vi "Lab Panel V5.0.vi"() -> ()   [LabVIEW 2013] (continued)
                      tunnel: w2173 -> [w2180 _]
                      tunnel: w2172 -> [w2179 _]
                      tunnel: w2171 -> [w2178 _]
                      frame True {
                        n1199 = stacked-sequence {
                          tunnel: w2180 -> [w2183 _]
                          tunnel: w2179 -> [_ w2188]
                          tunnel: w2178 -> [w2181 _]
                          frame #0 {
                            n1200 = Build Array("T-RISE") -> (w2185:string[])
                            n1201 = Build Array(w2183) -> (w2184:dbl[])
                            n1202 = TDMS Write(0:w2181, 5:"TEST PASS", 7:w2185, 9:w2184) -> (15:w2187:errorcluster)  [unwired: 2 in, 3 out]
                            n1203 = local write "data file error"(w2187) -> ()
                          }
                          frame #1 {
                            n1204 = Bundle(cluster=w2188, "STATUS"="T-RISE PASS") -> (w2190:T4)  [unwired: 2 in]
                            n1205 = local write "RESULT LAB01-1"(TRUE) -> ()
                            n1206 = local write "DISP LAB01-1"(w2190) -> ()
                          }
                        }
                      }
                      frame False {
                      }
                    }
                  }
                }
              }
              frame #1 {
                # "LAB01-2"
                n1207 = Equal?(x=w2193, y=2) -> (x = y?=w2196:bool)
                n1208 = local read "DISP LAB01-2"() -> (w2198:T4)
                n1209 = Unbundle(w2198) -> ("STATUS"=w2199:string)  [unwired: 2 out]
                n1210 = Equal?(x=w2199, y="RUN") -> (x = y?=w2195:bool)
                n1211 = And(x=w2195, y=w2196) -> (x .and. y?=w2194:bool)
                n1212 = case shown="True" w2194 {
                  tunnel: w2198 -> [_ w2202]
                  tunnel: w2192 -> [_ w2205]
                  frame False {
                  }
                  frame True {
                    n1213 = local read "SET LAB01-2"() -> (w2204:T5)
                    n1214 = local read "TDMS LAB01-2"() -> (w2201:refnum<k34>)
                    n1215 = Unbundle(w2202) -> ("CYCLE"=w2206:dbl)  [unwired: 2 out]
                    n1216 = Unbundle(w2204) -> ("T-RISE mins"=w2203:dbl)  [unwired: 4 out]
                    n1217 = Greater Or Equal?(x=w2206, y=w2205) -> (x >= y?=w2207:bool)
                    n1218 = case shown="True" w2207 {
                      tunnel: w2203 -> [w2210 _]
                      tunnel: w2202 -> [w2209 _]
                      tunnel: w2201 -> [w2208 _]
                      frame True {
                        n1219 = stacked-sequence {
                          tunnel: w2210 -> [w2213 _]
                          tunnel: w2209 -> [_ w2218]
                          tunnel: w2208 -> [w2211 _]
                          frame #0 {
                            n1220 = Build Array("T-RISE") -> (w2215:string[])
                            n1221 = Build Array(w2213) -> (w2214:dbl[])
                            n1222 = TDMS Write(0:w2211, 5:"TEST PASS", 7:w2215, 9:w2214) -> (15:w2217:errorcluster)  [unwired: 2 in, 3 out]
                            n1223 = local write "data file error"(w2217) -> ()
                          }
                          frame #1 {
                            n1224 = Bundle(cluster=w2218, "STATUS"="T-RISE PASS") -> (w2220:T4)  [unwired: 2 in]
                            n1225 = local write "RESULT LAB01-2"(TRUE) -> ()
                            n1226 = local write "DISP LAB01-2"(w2220) -> ()
                          }
                        }
                      }
                      frame False {
                      }
                    }
                  }
                }
              }
              frame #2 {
                # "LAB02-1"
                n1227 = Equal?(x=w2223, y=2) -> (x = y?=w2226:bool)
                n1228 = local read "DISP LAB02-1"() -> (w2228:T4)
                n1229 = Unbundle(w2228) -> ("STATUS"=w2229:string)  [unwired: 2 out]
                n1230 = Equal?(x=w2229, y="RUN") -> (x = y?=w2225:bool)
                n1231 = And(x=w2225, y=w2226) -> (x .and. y?=w2224:bool)
                n1232 = case shown="True" w2224 {
                  tunnel: w2228 -> [_ w2232]
                  tunnel: w2222 -> [_ w2235]
                  frame False {
                  }
                  frame True {
                    n1233 = local read "SET LAB02-1"() -> (w2234:T5)
                    n1234 = local read "TDMS LAB02-1"() -> (w2231:refnum<k34>)
                    n1235 = Unbundle(w2232) -> ("CYCLE"=w2236:dbl)  [unwired: 2 out]
                    n1236 = Unbundle(w2234) -> ("T-RISE mins"=w2233:dbl)  [unwired: 4 out]
                    n1237 = Greater Or Equal?(x=w2236, y=w2235) -> (x >= y?=w2237:bool)
                    n1238 = case shown="True" w2237 {
                      tunnel: w2233 -> [w2240 _]
                      tunnel: w2232 -> [w2239 _]
                      tunnel: w2231 -> [w2238 _]
                      frame True {
                        n1239 = stacked-sequence {
                          tunnel: w2240 -> [w2243 _]
                          tunnel: w2239 -> [_ w2248]
                          tunnel: w2238 -> [w2241 _]
                          frame #0 {
                            n1240 = Build Array("T-RISE") -> (w2245:string[])
                            n1241 = Build Array(w2243) -> (w2244:dbl[])
                            n1242 = TDMS Write(0:w2241, 5:"TEST PASS", 7:w2245, 9:w2244) -> (15:w2247:errorcluster)  [unwired: 2 in, 3 out]
                            n1243 = local write "data file error"(w2247) -> ()
                          }
                          frame #1 {
                            n1244 = Bundle(cluster=w2248, "STATUS"="T-RISE PASS") -> (w2250:T4)  [unwired: 2 in]
                            n1245 = local write "RESULT LAB02-1"(TRUE) -> ()
                            n1246 = local write "DISP LAB02-1"(w2250) -> ()
                          }
                        }
                      }
                      frame False {
                      }
                    }
                  }
                }
              }
              frame #3 {
                # "LAB02-2"
                n1247 = Equal?(x=w2253, y=2) -> (x = y?=w2256:bool)
                n1248 = local read "DISP LAB02-2"() -> (w2258:T4)
                n1249 = Unbundle(w2258) -> ("STATUS"=w2259:string)  [unwired: 2 out]
                n1250 = Equal?(x=w2259, y="RUN") -> (x = y?=w2255:bool)
                n1251 = And(x=w2255, y=w2256) -> (x .and. y?=w2254:bool)
                n1252 = case shown="True" w2254 {
                  tunnel: w2258 -> [_ w2262]
                  tunnel: w2252 -> [_ w2265]
                  frame False {
                  }
                  frame True {
                    n1253 = local read "SET LAB02-2"() -> (w2264:T5)
                    n1254 = local read "TDMS LAB02-2"() -> (w2261:refnum<k34>)
                    n1255 = Unbundle(w2262) -> ("CYCLE"=w2266:dbl)  [unwired: 2 out]
                    n1256 = Unbundle(w2264) -> ("T-RISE mins"=w2263:dbl)  [unwired: 4 out]
                    n1257 = Greater Or Equal?(x=w2266, y=w2265) -> (x >= y?=w2267:bool)
                    n1258 = case shown="True" w2267 {
                      tunnel: w2263 -> [w2270 _]
                      tunnel: w2262 -> [w2269 _]
                      tunnel: w2261 -> [w2268 _]
                      frame True {
                        n1259 = stacked-sequence {
                          tunnel: w2270 -> [w2273 _]
                          tunnel: w2269 -> [_ w2278]
                          tunnel: w2268 -> [w2271 _]
                          frame #0 {
                            n1260 = Build Array("T-RISE") -> (w2275:string[])
                            n1261 = Build Array(w2273) -> (w2274:dbl[])
                            n1262 = TDMS Write(0:w2271, 5:"TEST PASS", 7:w2275, 9:w2274) -> (15:w2277:errorcluster)  [unwired: 2 in, 3 out]
                            n1263 = local write "data file error"(w2277) -> ()
                          }
                          frame #1 {
                            n1264 = Bundle(cluster=w2278, "STATUS"="T-RISE PASS") -> (w2280:T4)  [unwired: 2 in]
                            n1265 = local write "RESULT LAB02-2"(TRUE) -> ()
                            n1266 = local write "DISP LAB02-2"(w2280) -> ()
                          }
                        }
                      }
                      frame False {
                      }
                    }
                  }
                }
              }
              frame #4 {
                # "LAB03-1"
                n1267 = Equal?(x=w2283, y=2) -> (x = y?=w2286:bool)
                n1268 = local read "DISP LAB03-1"() -> (w2288:T4)
                n1269 = Unbundle(w2288) -> ("STATUS"=w2289:string)  [unwired: 2 out]
                n1270 = Equal?(x=w2289, y="RUN") -> (x = y?=w2285:bool)
                n1271 = And(x=w2285, y=w2286) -> (x .and. y?=w2284:bool)
                n1272 = case shown="True" w2284 {
                  tunnel: w2288 -> [_ w2292]
                  tunnel: w2282 -> [_ w2295]
                  frame False {
                  }
                  frame True {
                    n1273 = local read "SET LAB03-1"() -> (w2294:T5)
                    n1274 = local read "TDMS LAB03-1"() -> (w2291:refnum<k34>)
                    n1275 = Unbundle(w2292) -> ("CYCLE"=w2296:dbl)  [unwired: 2 out]
                    n1276 = Unbundle(w2294) -> ("T-RISE mins"=w2293:dbl)  [unwired: 4 out]
                    n1277 = Greater Or Equal?(x=w2296, y=w2295) -> (x >= y?=w2297:bool)
                    n1278 = case shown="True" w2297 {
                      tunnel: w2293 -> [w2300 _]
                      tunnel: w2292 -> [w2299 _]
                      tunnel: w2291 -> [w2298 _]
                      frame True {
                        n1279 = stacked-sequence {
                          tunnel: w2300 -> [w2303 _]
                          tunnel: w2299 -> [_ w2308]
                          tunnel: w2298 -> [w2301 _]
                          frame #0 {
                            n1280 = Build Array("T-RISE") -> (w2305:string[])
                            n1281 = Build Array(w2303) -> (w2304:dbl[])
                            n1282 = TDMS Write(0:w2301, 5:"TEST PASS", 7:w2305, 9:w2304) -> (15:w2307:errorcluster)  [unwired: 2 in, 3 out]
                            n1283 = local write "data file error"(w2307) -> ()
                          }
                          frame #1 {
                            n1284 = Bundle(cluster=w2308, "STATUS"="T-RISE PASS") -> (w2310:T4)  [unwired: 2 in]
                            n1285 = local write "RESULT LAB03-1"(TRUE) -> ()
                            n1286 = local write "DISP LAB03-1"(w2310) -> ()
                          }
                        }
                      }
                      frame False {
                      }
                    }
                  }
                }
              }
              frame #5 {
                # "LAB03-2"
                n1287 = Equal?(x=w2313, y=2) -> (x = y?=w2316:bool)
                n1288 = local read "DISP LAB03-2"() -> (w2318:T4)
                n1289 = Unbundle(w2318) -> ("STATUS"=w2319:string)  [unwired: 2 out]
                n1290 = Equal?(x=w2319, y="RUN") -> (x = y?=w2315:bool)
                n1291 = And(x=w2315, y=w2316) -> (x .and. y?=w2314:bool)
                n1292 = case shown="True" w2314 {
                  tunnel: w2318 -> [_ w2322]
                  tunnel: w2312 -> [_ w2325]
                  frame False {
                  }
                  frame True {
                    n1293 = local read "SET LAB03-2"() -> (w2324:T5)
                    n1294 = local read "TDMS LAB03-2"() -> (w2321:refnum<k34>)
                    n1295 = Unbundle(w2322) -> ("CYCLE"=w2326:dbl)  [unwired: 2 out]
                    n1296 = Unbundle(w2324) -> ("T-RISE mins"=w2323:dbl)  [unwired: 4 out]
                    n1297 = Greater Or Equal?(x=w2326, y=w2325) -> (x >= y?=w2327:bool)
                    n1298 = case shown="True" w2327 {
                      tunnel: w2323 -> [w2330 _]
                      tunnel: w2322 -> [w2329 _]
                      tunnel: w2321 -> [w2328 _]
                      frame True {
                        n1299 = stacked-sequence {
                          tunnel: w2330 -> [w2333 _]
                          tunnel: w2329 -> [_ w2338]
                          tunnel: w2328 -> [w2331 _]
                          frame #0 {
                            n1300 = Build Array("T-RISE") -> (w2335:string[])
                            n1301 = Build Array(w2333) -> (w2334:dbl[])
                            n1302 = TDMS Write(0:w2331, 5:"TEST PASS", 7:w2335, 9:w2334) -> (15:w2337:errorcluster)  [unwired: 2 in, 3 out]
                            n1303 = local write "data file error"(w2337) -> ()
                          }
                          frame #1 {
                            n1304 = Bundle(cluster=w2338, "STATUS"="T-RISE PASS") -> (w2340:T4)  [unwired: 2 in]
                            n1305 = local write "RESULT LAB03-2"(TRUE) -> ()
                            n1306 = local write "DISP LAB03-2"(w2340) -> ()
                          }
                        }
                      }
                      frame False {
                      }
                    }
                  }
                }
              }
              frame #6 {
                # "LAB04-1"
                n1307 = Equal?(x=w2343, y=2) -> (x = y?=w2346:bool)
                n1308 = local read "DISP LAB04-1"() -> (w2348:T4)
                n1309 = Unbundle(w2348) -> ("STATUS"=w2349:string)  [unwired: 2 out]
                n1310 = Equal?(x=w2349, y="RUN") -> (x = y?=w2345:bool)
                n1311 = And(x=w2345, y=w2346) -> (x .and. y?=w2344:bool)
                n1312 = case shown="True" w2344 {
                  tunnel: w2348 -> [_ w2352]
                  tunnel: w2342 -> [_ w2355]
                  frame False {
                  }
                  frame True {
                    n1313 = local read "SET LAB04-1"() -> (w2354:T5)
                    n1314 = local read "TDMS LAB04-1"() -> (w2351:refnum<k34>)
                    n1315 = Unbundle(w2352) -> ("CYCLE"=w2356:dbl)  [unwired: 2 out]
                    n1316 = Unbundle(w2354) -> ("T-RISE mins"=w2353:dbl)  [unwired: 4 out]
                    n1317 = Greater Or Equal?(x=w2356, y=w2355) -> (x >= y?=w2357:bool)
                    n1318 = case shown="True" w2357 {
                      tunnel: w2353 -> [w2360 _]
                      tunnel: w2352 -> [w2359 _]
                      tunnel: w2351 -> [w2358 _]
                      frame True {
                        n1319 = stacked-sequence {
                          tunnel: w2360 -> [w2363 _]
                          tunnel: w2359 -> [_ w2368]
                          tunnel: w2358 -> [w2361 _]
                          frame #0 {
                            n1320 = Build Array("T-RISE") -> (w2365:string[])
                            n1321 = Build Array(w2363) -> (w2364:dbl[])
                            n1322 = TDMS Write(0:w2361, 5:"TEST PASS", 7:w2365, 9:w2364) -> (15:w2367:errorcluster)  [unwired: 2 in, 3 out]
                            n1323 = local write "data file error"(w2367) -> ()
                          }
                          frame #1 {
                            n1324 = Bundle(cluster=w2368, "STATUS"="T-RISE PASS") -> (w2370:T4)  [unwired: 2 in]
                            n1325 = local write "RESULT LAB04-1"(TRUE) -> ()
                            n1326 = local write "DISP LAB04-1"(w2370) -> ()
                          }
                        }
                      }
                      frame False {
                      }
                    }
                  }
                }
              }
              frame #7 {
                # "LAB04-2"
                n1327 = Equal?(x=w2373, y=2) -> (x = y?=w2376:bool)
                n1328 = local read "DISP LAB04-2"() -> (w2378:T4)
                n1329 = Unbundle(w2378) -> ("STATUS"=w2379:string)  [unwired: 2 out]
                n1330 = Equal?(x=w2379, y="RUN") -> (x = y?=w2375:bool)
                n1331 = And(x=w2375, y=w2376) -> (x .and. y?=w2374:bool)
                n1332 = case shown="True" w2374 {
                  tunnel: w2378 -> [_ w2382]
                  tunnel: w2372 -> [_ w2385]
                  frame False {
                  }
                  frame True {
                    n1333 = local read "SET LAB04-2"() -> (w2384:T5)
                    n1334 = local read "TDMS LAB04-2"() -> (w2381:refnum<k34>)
                    n1335 = Unbundle(w2382) -> ("CYCLE"=w2386:dbl)  [unwired: 2 out]
                    n1336 = Unbundle(w2384) -> ("T-RISE mins"=w2383:dbl)  [unwired: 4 out]
                    n1337 = Greater Or Equal?(x=w2386, y=w2385) -> (x >= y?=w2387:bool)
                    n1338 = case shown="True" w2387 {
                      tunnel: w2383 -> [w2390 _]
                      tunnel: w2382 -> [w2389 _]
                      tunnel: w2381 -> [w2388 _]
                      frame True {
                        n1339 = stacked-sequence {
                          tunnel: w2390 -> [w2393 _]
                          tunnel: w2389 -> [_ w2398]
                          tunnel: w2388 -> [w2391 _]
                          frame #0 {
                            n1340 = Build Array("T-RISE") -> (w2395:string[])
                            n1341 = Build Array(w2393) -> (w2394:dbl[])
                            n1342 = TDMS Write(0:w2391, 5:"TEST PASS", 7:w2395, 9:w2394) -> (15:w2397:errorcluster)  [unwired: 2 in, 3 out]
                            n1343 = local write "data file error"(w2397) -> ()
                          }
                          frame #1 {
                            n1344 = Bundle(cluster=w2398, "STATUS"="T-RISE PASS") -> (w2400:T4)  [unwired: 2 in]
                            n1345 = local write "RESULT LAB04-2"(TRUE) -> ()
                            n1346 = local write "DISP LAB04-2"(w2400) -> ()
                          }
                        }
                      }
                      frame False {
                      }
                    }
                  }
                }
              }
              frame #8 {
                # "LAB05-1"
                n1347 = Equal?(x=w2403, y=2) -> (x = y?=w2406:bool)
                n1348 = local read "DISP LAB05-1"() -> (w2408:T4)
                n1349 = Unbundle(w2408) -> ("STATUS"=w2409:string)  [unwired: 2 out]
                n1350 = Equal?(x=w2409, y="RUN") -> (x = y?=w2405:bool)
                n1351 = And(x=w2405, y=w2406) -> (x .and. y?=w2404:bool)
                n1352 = case shown="True" w2404 {
                  tunnel: w2408 -> [_ w2412]
                  tunnel: w2402 -> [_ w2415]
                  frame False {
                  }
                  frame True {
                    n1353 = local read "SET LAB05-1"() -> (w2414:T5)
                    n1354 = local read "TDMS LAB05-1"() -> (w2411:refnum<k34>)
                    n1355 = Unbundle(w2412) -> ("CYCLE"=w2416:dbl)  [unwired: 2 out]
                    n1356 = Unbundle(w2414) -> ("T-RISE mins"=w2413:dbl)  [unwired: 4 out]
                    n1357 = Greater Or Equal?(x=w2416, y=w2415) -> (x >= y?=w2417:bool)
                    n1358 = case shown="True" w2417 {
                      tunnel: w2413 -> [w2420 _]
                      tunnel: w2412 -> [w2419 _]
                      tunnel: w2411 -> [w2418 _]
                      frame True {
                        n1359 = stacked-sequence {
                          tunnel: w2420 -> [w2423 _]
                          tunnel: w2419 -> [_ w2428]
                          tunnel: w2418 -> [w2421 _]
                          frame #0 {
                            n1360 = Build Array("T-RISE") -> (w2425:string[])
                            n1361 = Build Array(w2423) -> (w2424:dbl[])
                            n1362 = TDMS Write(0:w2421, 5:"TEST PASS", 7:w2425, 9:w2424) -> (15:w2427:errorcluster)  [unwired: 2 in, 3 out]
                            n1363 = local write "data file error"(w2427) -> ()
                          }
                          frame #1 {
                            n1364 = Bundle(cluster=w2428, "STATUS"="T-RISE PASS") -> (w2430:T4)  [unwired: 2 in]
                            n1365 = local write "RESULT LAB05-1"(TRUE) -> ()
                            n1366 = local write "DISP LAB05-1"(w2430) -> ()
                          }
                        }
                      }
                      frame False {
                      }
                    }
                  }
                }
              }
              frame #9 {
                # "LAB05-2"
                n1367 = Equal?(x=w2433, y=2) -> (x = y?=w2436:bool)
                n1368 = local read "DISP LAB05-2"() -> (w2438:T4)
                n1369 = Unbundle(w2438) -> ("STATUS"=w2439:string)  [unwired: 2 out]
                n1370 = Equal?(x=w2439, y="RUN") -> (x = y?=w2435:bool)
                n1371 = And(x=w2435, y=w2436) -> (x .and. y?=w2434:bool)
                n1372 = case shown="True" w2434 {
                  tunnel: w2438 -> [_ w2442]
                  tunnel: w2432 -> [_ w2445]
                  frame False {
                  }
                  frame True {
                    n1373 = local read "SET LAB05-2"() -> (w2444:T5)
                    n1374 = local read "TDMS LAB05-2"() -> (w2441:refnum<k34>)
                    n1375 = Unbundle(w2442) -> ("CYCLE"=w2446:dbl)  [unwired: 2 out]
                    n1376 = Unbundle(w2444) -> ("T-RISE mins"=w2443:dbl)  [unwired: 4 out]
                    n1377 = Greater Or Equal?(x=w2446, y=w2445) -> (x >= y?=w2447:bool)
                    n1378 = case shown="True" w2447 {
                      tunnel: w2443 -> [w2450 _]
                      tunnel: w2442 -> [w2449 _]
                      tunnel: w2441 -> [w2448 _]
                      frame True {
                        n1379 = stacked-sequence {
                          tunnel: w2450 -> [w2453 _]
                          tunnel: w2449 -> [_ w2458]
                          tunnel: w2448 -> [w2451 _]
                          frame #0 {
                            n1380 = Build Array("T-RISE") -> (w2455:string[])
                            n1381 = Build Array(w2453) -> (w2454:dbl[])
                            n1382 = TDMS Write(0:w2451, 5:"TEST PASS", 7:w2455, 9:w2454) -> (15:w2457:errorcluster)  [unwired: 2 in, 3 out]
                            n1383 = local write "data file error"(w2457) -> ()
                          }
                          frame #1 {
                            n1384 = Bundle(cluster=w2458, "STATUS"="T-RISE PASS") -> (w2460:T4)  [unwired: 2 in]
                            n1385 = local write "RESULT LAB05-2"(TRUE) -> ()
                            n1386 = local write "DISP LAB05-2"(w2460) -> ()
                          }
                        }
                      }
                      frame False {
                      }
                    }
                  }
                }
              }
            }
          }
          frame #6 {
            # "end test & close test files"
            n1387 = stacked-sequence {
              tunnel: w2471 -> [_ _ _ _ _ _ _ _ _ _]
              tunnel: w2472 -> [_ _ _ _ _ _ _ _ _ _]
              tunnel: w2470 -> [_ _ _ _ _ _ _ _ _ _]
              tunnel: w2469 -> [_ _ _ _ _ _ _ _ _ _]
              tunnel: w2468 -> [_ _ _ _ _ _ _ _ _ _]
              tunnel: w2467 -> [_ _ _ _ _ _ _ _ _ _]
              tunnel: w2466 -> [_ _ _ _ _ _ _ _ _ _]
              tunnel: w2465 -> [_ _ _ _ _ _ _ _ _ _]
              tunnel: w2464 -> [_ _ _ _ _ _ _ _ _ _]
              tunnel: w2463 -> [_ _ _ _ _ _ _ _ _ _]
              frame #0 {
                # "LAB01-1"
                n1388 = local read "DISP LAB01-1"() -> (w2476:T4)
                n1389 = local read "run lab01-1"() -> (w2473:bool)
                n1390 = local read "TDMS LAB01-1"() -> (w2474:refnum<k34>)
                n1391 = Unbundle(w2476) -> ("CYCLE"=w2477:dbl, "STATUS"=w2475:string)  [unwired: 1 out]
                n1392 = case shown="True" w2473 {
                  tunnel: w2477 -> [_ w2478]
                  tunnel: w2476 -> [_ w2481]
                  tunnel: w2475 -> [_ w2480]
                  tunnel: w2474 -> [_ w2479]
                  frame False {
                  }
                  frame True {
                    n1393 = Not Equal?(x=w2480, y="RUN") -> (x != y?=w2482:bool)
                    n1394 = Greater?(x=w2478, y=2.0) -> (0:w2484:bool)
                    n1395 = And(x=w2484, y=w2482) -> (x .and. y?=w2483:bool)
                    n1396 = case shown="True" w2483 {
                      tunnel: w2481 -> [_ w2489]
                      tunnel: w2479 -> [_ w2488]
                      tunnel: w2478 -> [_ w2487]
                      frame False {
                      }
                      frame True {
                        n1397 = stacked-sequence {
                          tunnel: w2489 -> [w2493 _ _]
                          tunnel: w2488 -> [_ w2495 _]
                          tunnel: w2487 -> [_ _ _]
                          frame #0 {
                            w2490 = FALSE
                            n1398 = local write "mail control"("END") -> ()
                            n1399 = Bundle(cluster=w2493) -> (w2492:T4)  [unwired: 3 in]
                            n1400 = local write "DISP LAB01-1"(w2492) -> ()
                            n1401 = local write "O/I  LAB01-1"(w2490) -> ()
                            n1402 = local write "run lab01-1"(w2490) -> ()
                            n1403 = local write "RUN LAB01-1"(w2490) -> ()
                          }
                          frame #1 {
                            n1404 = TDMS Close(11:w2495) -> (0:w2494:errorcluster)  [unwired: 1 in, 1 out]
                            n1405 = local write "data file error"(w2494) -> ()
                          }
                          frame #2 {
                            n1406 = stacked-sequence {
                              tunnel: "LAB01-1" -> [w2498 w2500]
                              frame #0 {
                                n1407 = call "sub vi - defrag tdms v1.vi"("panel id"=w2498) -> ("error out"=w2497:errorcluster)  [unwired: 10 in]
                                n1408 = local write "data file error"(w2497) -> ()
                              }
                              frame #1 {
                                n1409 = call "Save data file to network drive v2.vi"("panel id"=w2500) -> ("network file save error"=w2499:errorcluster)  [unwired: 9 in, 1 out]
                                n1410 = local write "data file error"(w2499) -> ()
                              }
                            }
                          }
                        }
                      }
                    }
                  }
                }
              }
              frame #1 {
                # "LAB01-2"
                n1411 = local read "run lab01-2"() -> (w2501:bool)
                n1412 = case shown="True" w2501 {
                  frame False {
                  }
                  frame True {
                    n1413 = local read "DISP LAB01-2"() -> (w2508:T4)
                    n1414 = local read "TDMS LAB01-2"() -> (w2507:refnum<k34>)
                    n1415 = Unbundle(w2508) -> ("CYCLE"=w2502:dbl, "STATUS"=w2509:string)  [unwired: 1 out]
                    n1416 = Not Equal?(x=w2509, y="RUN") -> (x != y?=w2504:bool)
                    n1417 = Greater?(x=w2502, y=2.0) -> (0:w2505:bool)
                    n1418 = And(x=w2505, y=w2504) -> (x .and. y?=w2503:bool)
                    n1419 = case shown="True" w2503 {
                      tunnel: w2508 -> [_ w2513]
                      tunnel: w2507 -> [_ w2512]
                      tunnel: w2502 -> [_ w2511]
                      frame False {
                      }
                      frame True {
                        n1420 = stacked-sequence {
                          tunnel: w2513 -> [w2516 _ _]
                          tunnel: w2512 -> [_ w2518 _]
                          tunnel: w2511 -> [_ _ _]
                          frame #0 {
                            w2514 = FALSE
                            n1421 = local write "mail control"("END") -> ()
                            n1422 = Bundle(cluster=w2516) -> (w2517:T4)  [unwired: 3 in]
                            n1423 = local write "RUN LAB01-2"(w2514) -> ()
                            n1424 = local write "run lab01-2"(w2514) -> ()
                            n1425 = local write "O/I  LAB01-2"(w2514) -> ()
                            n1426 = local write "DISP LAB01-2"(w2517) -> ()
                          }
                          frame #1 {
                            n1427 = TDMS Close(11:w2518) -> (0:w2519:errorcluster)  [unwired: 1 in, 1 out]
                            n1428 = local write "data file error"(w2519) -> ()
                          }
                          frame #2 {
                            n1429 = stacked-sequence {
                              tunnel: "LAB01-2" -> [w2522 w2524]
                              frame #0 {
                                n1430 = call "sub vi - defrag tdms v1.vi"("panel id"=w2522) -> ("error out"=w2521:errorcluster)  [unwired: 10 in]
                                n1431 = local write "data file error"(w2521) -> ()
                              }
                              frame #1 {
                                n1432 = call "Save data file to network drive v2.vi"("panel id"=w2524) -> ("network file save error"=w2523:errorcluster)  [unwired: 9 in, 1 out]
                                n1433 = local write "data file error"(w2523) -> ()
                              }
                            }
                          }
                        }
                      }
                    }
                  }
                }
              }
              frame #2 {
                # "LAB02-1"
                n1434 = local read "run lab02-1"() -> (w2525:bool)
                n1435 = case shown="True" w2525 {
                  frame False {
                  }
                  frame True {
                    n1436 = local read "DISP LAB02-1"() -> (w2532:T4)
                    n1437 = Unbundle(w2532) -> ("CYCLE"=w2528:dbl, "STATUS"=w2533:string)  [unwired: 1 out]
                    n1438 = local read "TDMS LAB02-1"() -> (w2531:refnum<k34>)
                    n1439 = Not Equal?(x=w2533, y="RUN") -> (x != y?=w2527:bool)
                    n1440 = Greater?(x=w2528, y=2.0) -> (0:w2529:bool)
                    n1441 = And(x=w2529, y=w2527) -> (x .and. y?=w2526:bool)
                    n1442 = case shown="True" w2526 {
                      tunnel: w2532 -> [_ w2536]
                      tunnel: w2531 -> [_ w2535]
                      frame False {
                      }
                      frame True {
                        n1443 = stacked-sequence {
                          tunnel: w2536 -> [w2539 _ _]
                          tunnel: w2535 -> [_ w2541 _]
                          frame #0 {
                            w2537 = FALSE
                            n1444 = local write "mail control"("END") -> ()
                            n1445 = Bundle(cluster=w2539) -> (w2540:T4)  [unwired: 3 in]
                            n1446 = local write "O/I  LAB02-1"(w2537) -> ()
                            n1447 = local write "RUN LAB02-1"(w2537) -> ()
                            n1448 = local write "run lab02-1"(w2537) -> ()
                            n1449 = local write "DISP LAB02-1"(w2540) -> ()
                          }
                          frame #1 {
                            n1450 = TDMS Close(11:w2541) -> (0:w2542:errorcluster)  [unwired: 1 in, 1 out]
                            n1451 = local write "data file error"(w2542) -> ()
                          }
                          frame #2 {
                            n1452 = stacked-sequence {
                              tunnel: "LAB02-1" -> [w2545 w2547]
                              frame #0 {
                                n1453 = call "sub vi - defrag tdms v1.vi"("panel id"=w2545) -> ("error out"=w2544:errorcluster)  [unwired: 10 in]
                                n1454 = local write "data file error"(w2544) -> ()
                              }
                              frame #1 {
                                n1455 = call "Save data file to network drive v2.vi"("panel id"=w2547) -> ("network file save error"=w2546:errorcluster)  [unwired: 9 in, 1 out]
                                n1456 = local write "data file error"(w2546) -> ()
                              }
                            }
                          }
                        }
                      }
                    }
                  }
                }
              }
              frame #3 {
                # "LAB02-2"
                n1457 = local read "run lab02-2"() -> (w2548:bool)
                n1458 = case shown="True" w2548 {
                  frame False {
                  }
                  frame True {
                    n1459 = local read "DISP LAB02-2"() -> (w2555:T4)
                    n1460 = local read "TDMS LAB02-2"() -> (w2554:refnum<k34>)
                    n1461 = Unbundle(w2555) -> ("CYCLE"=w2551:dbl, "STATUS"=w2556:string)  [unwired: 1 out]
                    n1462 = Not Equal?(x=w2556, y="RUN") -> (x != y?=w2550:bool)
                    n1463 = Greater?(x=w2551, y=2.0) -> (0:w2552:bool)
                    n1464 = And(x=w2552, y=w2550) -> (x .and. y?=w2549:bool)
                    n1465 = case shown="True" w2549 {
                      tunnel: w2555 -> [_ w2559]
                      tunnel: w2554 -> [_ w2558]
                      frame False {
                      }
                      frame True {
                        n1466 = stacked-sequence {
                          tunnel: w2559 -> [w2562 _ _]
                          tunnel: w2558 -> [_ w2564 _]
                          frame #0 {
                            w2560 = FALSE
                            n1467 = local write "mail control"("END") -> ()
                            n1468 = Bundle(cluster=w2562) -> (w2563:T4)  [unwired: 3 in]
                            n1469 = local write "O/I  LAB02-2"(w2560) -> ()
                            n1470 = local write "run lab02-2"(w2560) -> ()
                            n1471 = local write "RUN LAB02-2"(w2560) -> ()
                            n1472 = local write "DISP LAB02-2"(w2563) -> ()
                          }
                          frame #1 {
                            n1473 = TDMS Close(11:w2564) -> (0:w2565:errorcluster)  [unwired: 1 in, 1 out]
                            n1474 = local write "data file error"(w2565) -> ()
                          }
                          frame #2 {
                            n1475 = stacked-sequence {
                              tunnel: "LAB02-2" -> [w2568 w2570]
                              frame #0 {
                                n1476 = call "sub vi - defrag tdms v1.vi"("panel id"=w2568) -> ("error out"=w2567:errorcluster)  [unwired: 10 in]
                                n1477 = local write "data file error"(w2567) -> ()
                              }
                              frame #1 {
                                n1478 = call "Save data file to network drive v2.vi"("panel id"=w2570) -> ("network file save error"=w2569:errorcluster)  [unwired: 9 in, 1 out]
                                n1479 = local write "data file error"(w2569) -> ()
                              }
                            }
                          }
                        }
                      }
                    }
                  }
                }
              }
              frame #4 {
                # "LAB03-1"
                n1480 = local read "run lab03-1"() -> (w2571:bool)
                n1481 = case shown="True" w2571 {
                  frame False {
                  }
                  frame True {
                    n1482 = local read "DISP LAB03-1"() -> (w2578:T4)
                    n1483 = local read "TDMS LAB03-1"() -> (w2577:refnum<k34>)
                    n1484 = Unbundle(w2578) -> ("CYCLE"=w2574:dbl, "STATUS"=w2579:string)  [unwired: 1 out]
                    n1485 = Not Equal?(x=w2579, y="RUN") -> (x != y?=w2573:bool)
                    n1486 = Greater?(x=w2574, y=2.0) -> (0:w2575:bool)
                    n1487 = And(x=w2575, y=w2573) -> (x .and. y?=w2572:bool)
                    n1488 = case shown="True" w2572 {
                      tunnel: w2578 -> [_ w2582]
                      tunnel: w2577 -> [_ w2581]
                      frame False {
                      }
                      frame True {
                        n1489 = stacked-sequence {
                          tunnel: w2582 -> [w2585 _ _]
                          tunnel: w2581 -> [_ w2587 _]
                          frame #0 {
                            w2583 = FALSE
                            n1490 = local write "mail control"("END") -> ()
                            n1491 = Bundle(cluster=w2585) -> (w2586:T4)  [unwired: 3 in]
                            n1492 = local write "O/I  LAB03-1"(w2583) -> ()
                            n1493 = local write "run lab03-1"(w2583) -> ()
                            n1494 = local write "RUN LAB03-1"(w2583) -> ()
                            n1495 = local write "DISP LAB03-1"(w2586) -> ()
                          }
                          frame #1 {
                            n1496 = TDMS Close(11:w2587) -> (0:w2588:errorcluster)  [unwired: 1 in, 1 out]
                            n1497 = local write "data file error"(w2588) -> ()
                          }
                          frame #2 {
                            n1498 = stacked-sequence {
                              tunnel: "LAB03-1" -> [w2591 w2593]
                              frame #0 {
                                n1499 = call "sub vi - defrag tdms v1.vi"("panel id"=w2591) -> ("error out"=w2590:errorcluster)  [unwired: 10 in]
                                n1500 = local write "data file error"(w2590) -> ()
                              }
                              frame #1 {
                                n1501 = call "Save data file to network drive v2.vi"("panel id"=w2593) -> ("network file save error"=w2592:errorcluster)  [unwired: 9 in, 1 out]
                                n1502 = local write "data file error"(w2592) -> ()
                              }
                            }
                          }
                        }
                      }
                    }
                  }
                }
              }
              frame #5 {
                # "LAB03-2"
                n1503 = local read "run lab03-2"() -> (w2594:bool)
                n1504 = case shown="True" w2594 {
                  frame False {
                  }
                  frame True {
                    n1505 = local read "DISP LAB03-2"() -> (w2601:T4)
                    n1506 = Unbundle(w2601) -> ("CYCLE"=w2597:dbl, "STATUS"=w2602:string)  [unwired: 1 out]
                    n1507 = local read "TDMS LAB03-2"() -> (w2600:refnum<k34>)
                    n1508 = Not Equal?(x=w2602, y="RUN") -> (x != y?=w2596:bool)
                    n1509 = Greater?(x=w2597, y=2.0) -> (0:w2598:bool)
                    n1510 = And(x=w2598, y=w2596) -> (x .and. y?=w2595:bool)
                    n1511 = case shown="True" w2595 {
                      tunnel: w2601 -> [_ w2605]
                      tunnel: w2600 -> [_ w2604]
                      frame False {
                      }
                      frame True {
                        n1512 = stacked-sequence {
                          tunnel: w2605 -> [w2608 _ _]
                          tunnel: w2604 -> [_ w2610 _]
                          frame #0 {
                            w2606 = FALSE
                            n1513 = local write "mail control"("END") -> ()
                            n1514 = Bundle(cluster=w2608) -> (w2609:T4)  [unwired: 3 in]
                            n1515 = local write "RUN LAB03-2"(w2606) -> ()
                            n1516 = local write "O/I  LAB03-2"(w2606) -> ()
                            n1517 = local write "DISP LAB03-2"(w2609) -> ()
                            n1518 = local write "run lab03-2"(w2606) -> ()
                          }
                          frame #1 {
                            n1519 = TDMS Close(11:w2610) -> (0:w2611:errorcluster)  [unwired: 1 in, 1 out]
                            n1520 = local write "data file error"(w2611) -> ()
                          }
                          frame #2 {
                            n1521 = stacked-sequence {
                              tunnel: "LAB03-2" -> [w2614 w2616]
                              frame #0 {
                                n1522 = call "sub vi - defrag tdms v1.vi"("panel id"=w2614) -> ("error out"=w2613:errorcluster)  [unwired: 10 in]
                                n1523 = local write "data file error"(w2613) -> ()
                              }
                              frame #1 {
                                n1524 = call "Save data file to network drive v2.vi"("panel id"=w2616) -> ("network file save error"=w2615:errorcluster)  [unwired: 9 in, 1 out]
                                n1525 = local write "data file error"(w2615) -> ()
                              }
                            }
                          }
                        }
                      }
                    }
                  }
                }
              }
              frame #6 {
                # "LAB04-1"
                n1526 = local read "run lab04-1"() -> (w2617:bool)
                n1527 = case shown="True" w2617 {
                  frame False {
                  }
                  frame True {
                    n1528 = local read "DISP LAB04-1"() -> (w2624:T4)
                    n1529 = Unbundle(w2624) -> ("CYCLE"=w2620:dbl, "STATUS"=w2625:string)  [unwired: 1 out]
                    n1530 = local read "TDMS LAB04-1"() -> (w2623:refnum<k34>)
                    n1531 = Not Equal?(x=w2625, y="RUN") -> (x != y?=w2619:bool)
                    n1532 = Greater?(x=w2620, y=2.0) -> (0:w2621:bool)
                    n1533 = And(x=w2621, y=w2619) -> (x .and. y?=w2618:bool)
                    n1534 = case shown="True" w2618 {
                      tunnel: w2624 -> [_ w2628]
                      tunnel: w2623 -> [_ w2627]
                      frame False {
                      }
                      frame True {
                        n1535 = stacked-sequence {
                          tunnel: w2628 -> [w2631 _ _]
                          tunnel: w2627 -> [_ w2633 _]
                          frame #0 {
                            w2629 = FALSE
                            n1536 = local write "mail control"("END") -> ()
                            n1537 = Bundle(cluster=w2631) -> (w2632:T4)  [unwired: 3 in]
                            n1538 = local write "RUN LAB04-1"(w2629) -> ()
                            n1539 = local write "O/I  LAB04-1"(w2629) -> ()
                            n1540 = local write "run lab04-1"(w2629) -> ()
                            n1541 = local write "DISP LAB04-1"(w2632) -> ()
                          }
                          frame #1 {
                            n1542 = TDMS Close(11:w2633) -> (0:w2634:errorcluster)  [unwired: 1 in, 1 out]
                            n1543 = local write "data file error"(w2634) -> ()
                          }
                          frame #2 {
                            n1544 = stacked-sequence {
                              tunnel: "LAB04-1" -> [w2637 w2639]
                              frame #0 {
                                n1545 = call "sub vi - defrag tdms v1.vi"("panel id"=w2637) -> ("error out"=w2636:errorcluster)  [unwired: 10 in]
                                n1546 = local write "data file error"(w2636) -> ()
                              }
                              frame #1 {
                                n1547 = call "Save data file to network drive v2.vi"("panel id"=w2639) -> ("network file save error"=w2638:errorcluster)  [unwired: 9 in, 1 out]
                                n1548 = local write "data file error"(w2638) -> ()
                              }
                            }
                          }
                        }
                      }
                    }
                  }
                }
              }
              frame #7 {
                # "LAB04-2"
                n1549 = local read "run lab04-2"() -> (w2640:bool)
                n1550 = case shown="True" w2640 {
                  frame False {
                  }
                  frame True {
                    n1551 = local read "DISP LAB04-2"() -> (w2647:T4)
                    n1552 = Unbundle(w2647) -> ("CYCLE"=w2643:dbl, "STATUS"=w2648:string)  [unwired: 1 out]
                    n1553 = Not Equal?(x=w2648, y="RUN") -> (x != y?=w2642:bool)
                    n1554 = local read "TDMS LAB04-2"() -> (w2646:refnum<k34>)
                    n1555 = Greater?(x=w2643, y=2.0) -> (0:w2644:bool)
                    n1556 = And(x=w2644, y=w2642) -> (x .and. y?=w2641:bool)
                    n1557 = case shown="True" w2641 {
                      tunnel: w2647 -> [_ w2651]
                      tunnel: w2646 -> [_ w2650]
                      frame False {
                      }
                      frame True {
                        n1558 = stacked-sequence {
                          tunnel: w2651 -> [w2654 _ _]
                          tunnel: w2650 -> [_ w2656 _]
                          frame #0 {
                            w2652 = FALSE
                            n1559 = local write "mail control"("END") -> ()
                            n1560 = Bundle(cluster=w2654) -> (w2655:T4)  [unwired: 3 in]
                            n1561 = local write "O/I  LAB04-2"(w2652) -> ()
                            n1562 = local write "RUN LAB04-2"(w2652) -> ()
                            n1563 = local write "run lab04-2"(w2652) -> ()
                            n1564 = local write "DISP LAB04-2"(w2655) -> ()
                          }
                          frame #1 {
                            n1565 = TDMS Close(11:w2656) -> (0:w2657:errorcluster)  [unwired: 1 in, 1 out]
                            n1566 = local write "data file error"(w2657) -> ()
                          }
                          frame #2 {
                            n1567 = stacked-sequence {
                              tunnel: "LAB04-2" -> [w2660 w2662]
                              frame #0 {
                                n1568 = call "sub vi - defrag tdms v1.vi"("panel id"=w2660) -> ("error out"=w2659:errorcluster)  [unwired: 10 in]
                                n1569 = local write "data file error"(w2659) -> ()
                              }
                              frame #1 {
                                n1570 = call "Save data file to network drive v2.vi"("panel id"=w2662) -> ("network file save error"=w2661:errorcluster)  [unwired: 9 in, 1 out]
                                n1571 = local write "data file error"(w2661) -> ()
                              }
                            }
                          }
                        }
                      }
                    }
                  }
                }
              }
              frame #8 {
                # "LAB05-1"
                n1572 = local read "run lab05-1"() -> (w2663:bool)
                n1573 = case shown="True" w2663 {
                  frame False {
                  }
                  frame True {
                    n1574 = local read "DISP LAB05-1"() -> (w2670:T4)
                    n1575 = Unbundle(w2670) -> ("CYCLE"=w2666:dbl, "STATUS"=w2671:string)  [unwired: 1 out]
                    n1576 = Not Equal?(x=w2671, y="RUN") -> (x != y?=w2665:bool)
                    n1577 = local read "TDMS LAB05-1"() -> (w2669:refnum<k34>)
                    n1578 = Greater?(x=w2666, y=2.0) -> (0:w2667:bool)
                    n1579 = And(x=w2667, y=w2665) -> (x .and. y?=w2664:bool)
                    n1580 = case shown="True" w2664 {
                      tunnel: w2670 -> [_ w2674]
